vi "SetConfig.vi"(8 "error in (no error)":errorcluster, 10 "PARAM":string, 11 "QuickControl in":refnum<class "QuickSilver.lvclass">) -> (0 "error out":errorcluster, 2 "RESP":string, 3 "QuickControl out":refnum<class "QuickSilver.lvclass">)   [LabVIEW 2018, in "QuickSilver.lvclass"]
uses:
  QuickSilver.lvclass
  QuickSilver.lvclass/QuickSilver.ctl
  <vilib>/Utility/config.llb/Write Key (String).vi
  <vilib>/Utility/config.llb/NI_LVConfig.lvlib
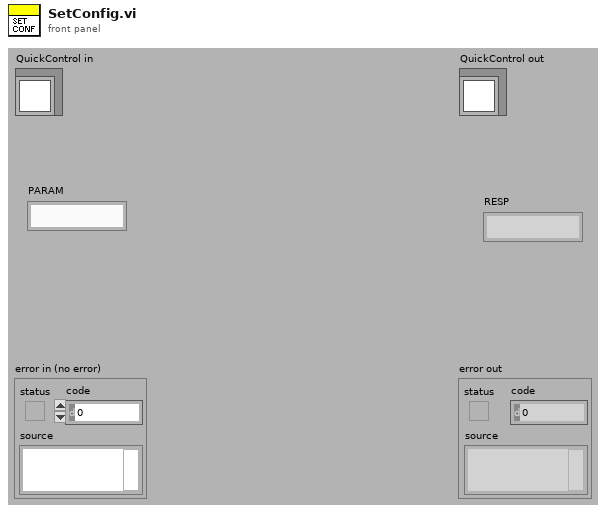
[diagram p1: front panel]
types:
  T1 = typedef "NI_LVConfig.lvlib/Config Data RefNum.ctl" = refnum<k1>
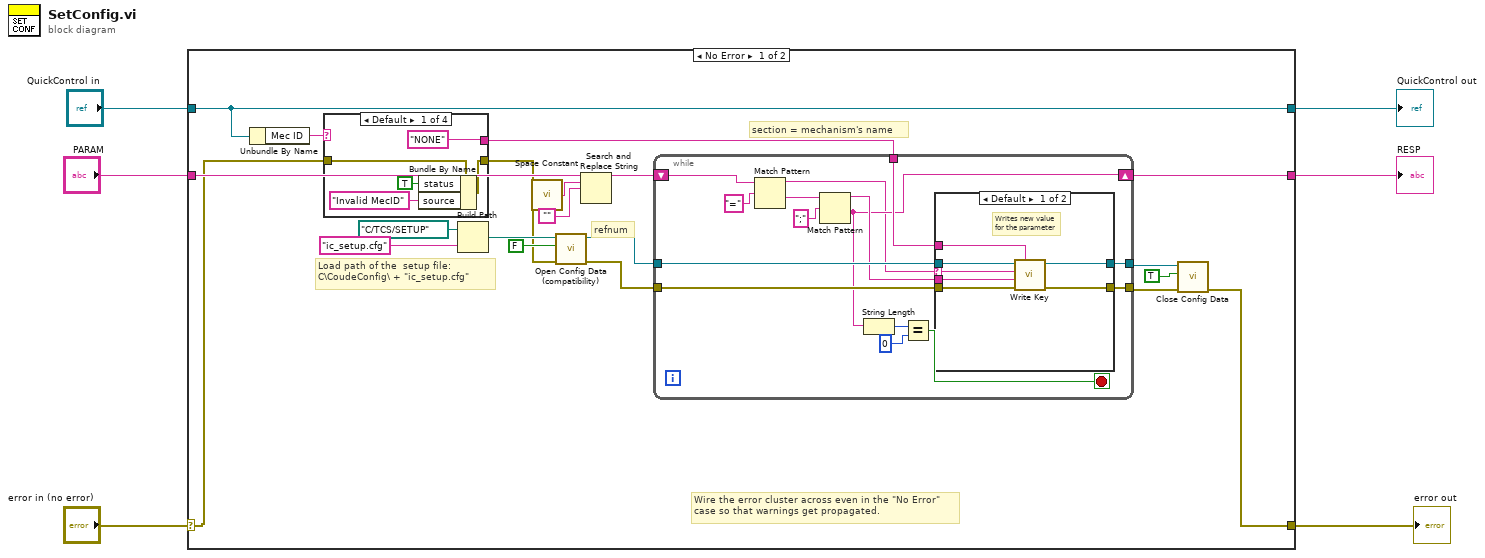
[diagram p0: block diagram]
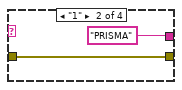
[diagram p2: hidden frame]
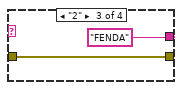
[diagram p3: hidden frame]
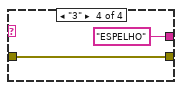
[diagram p4: hidden frame]
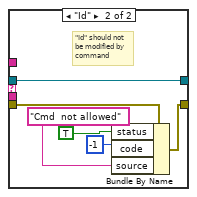
[diagram p5: hidden frame]
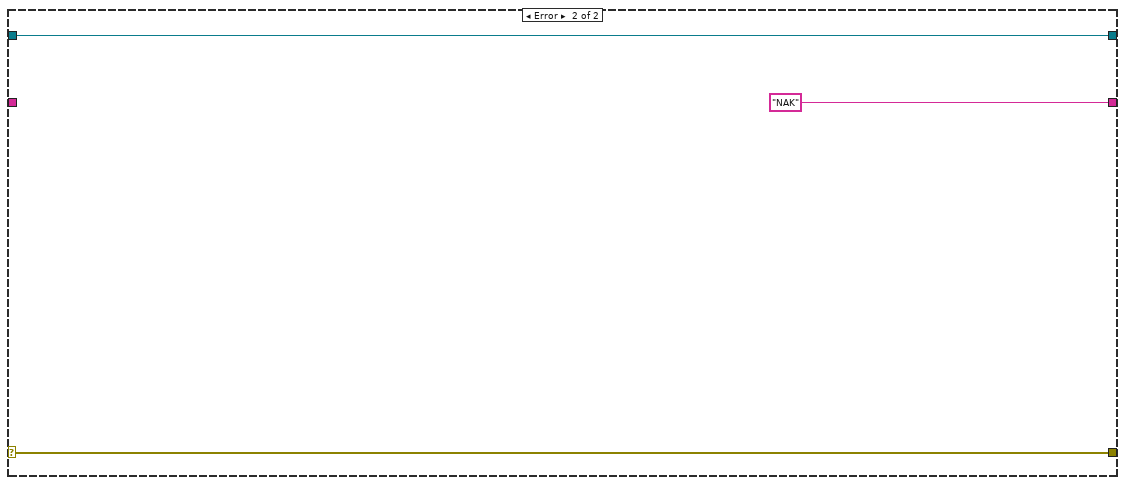
[diagram p6: hidden frame]
diagram:
  n1 = case shown="No Error" "error in (no error)" {
    selector: "error in (no error)" -> [w10 w68]
    tunnel: [w19 w68] -> w2
    tunnel: [w13 w67] -> w3
    tunnel: "QuickControl in" -> [w13 w67]
    tunnel: "PARAM" -> [w17 _]
    tunnel: [w8 "NAK" ("result string")] -> w1
    frame No Error {
      # "refnum"
      # "section = mechanism's name"
      # "Load path of the  setup file:\nC\\CoudeConfig\\ + \"ic_setup.cfg\""
      # "Wire the error cluster across even in the \"No Error\"\ncase so that warnings get propagated."
      n2 = Unbundle By Name(w13) -> ("Mec ID"=w12:string)
      n3 = case shown="Default" w12 {
        tunnel: ["NONE" "PRISMA" "FENDA" "ESPELHO"] -> w11
        tunnel: w10 -> [w30 w32 w34 w36]
        tunnel: [w29 w32 w34 w36] -> w9
        frame Default {
          n4 = Bundle By Name(cluster=w30, "status"=TRUE, "source"="Invalid MecID") -> (w29:errorcluster)
        }
        frame "1" {
        }
        frame "2" {
        }
        frame "3" {
        }
      }
      n5 = Build Path(base path=path "C:/TCS/SETUP", name or relative path="ic_setup.cfg") -> (appended path=w26:path)
      n6 = call <vilib>:"Space Constant.vi"() -> ("String"=w15:string)
      n7 = call <vilib>:"Open Config Data (compatibility).vi"("error in (no error)"=w9, "create file if necessary (T)"=FALSE ("create file if necessary? (T)"), "configuration file path"=w26) -> ("error out"=w22:errorcluster, "refnum"=w23:T1)  [unwired: 6 in, 1 out]
      n8 = Search and Replace String(input string=w17, search string=w15, replace string="") -> (result string=w16:string)  [unwired: 1 in, 7 out]
      n9 = while {
        tunnel: w23 -> [w52]
        tunnel: w22 -> [w51]
        tunnel: w11 -> [w50]
        shift-right: [w44] -> w8
        shift-left: w16 -> [w49]
        tunnel: [w42] -> w21
        tunnel: [w40] -> w20
        stop <- w39 stop-if-true
        n10 = Match Pattern(string=w49, regular expression="=") -> (before substring=w38:string, after substring=w47:string)  [unwired: 3 out]
        n11 = Match Pattern(string=w47, regular expression=";") -> (before substring=w45:string, after substring=w44:string)  [unwired: 3 out]
        n12 = String Length(string=w44) -> (length=w43:i32)
        n13 = Equal?(x=w43, y=0) -> (x = y?=w39:bool)
        n14 = case shown="Default" w38 {
          selector: w38 -> [w54 _]
          tunnel: w52 -> [w59 w65]
          tunnel: w51 -> [w58 w64]
          tunnel: w50 -> [w53 _]
          tunnel: w45 -> [w57 _]
          tunnel: [w56 w63] -> w42
          tunnel: [w55 w65] -> w40
          frame Default {
            # "Writes new value\nfor the parameter"
            n15 = call-poly <vilib>:"Write Key.vi"("section"=w53, "error in (no error)"=w58, "value"=w57, "key"=w54, "refnum"=w59) -> ("error out"=w56:errorcluster, "refnum out"=w55:T1)  [unwired: 1 in, 4 out]
          }
          frame "Id" {
            # "\"Id\" should not\nbe modified by \ncommand"
            n16 = Bundle By Name(cluster=w64, "status"=TRUE, "code"=-1, "source"="Cmd  not allowed") -> (w63:errorcluster)
          }
        }
      }
      n17 = call <vilib>:"Close Config Data.vi"("error in (no error)"=w21, "write file if changed (T)"=TRUE ("write configuration file? (T)"), "refnum"=w20) -> ("error out"=w19:errorcluster)  [unwired: 8 out]
    }
    frame Error {
    }
  }
  "error out" <- w2
  "QuickControl out" <- w3
  "RESP" <- w1
